vi "SGDA-Play Test.vi"(0 "StimChans":T1[](array[typedef]) {"Filter"."Stages"."IIR Filter"."Forward Coefficients" format="%.4f"; "Filter"."Stages"."IIR Filter"."Reverse Coefficients" format="%.4f"}, 1 "queue":refnum<queue>, 5 "Sampling rate (Hz)":dbl, 7 "Npts":i32, 11 "error in (no error)":errorcluster, 12 "Endpoint Config":T30[](array[typedef])) -> (15 "error out":errorcluster)   [LabVIEW 2020]
uses:
  Calibration VIs/Endpoint VIs/LV Source/Endpoint-Spec.ctl
  Calibration VIs/Endpoint VIs/LV Source/Endpoint-Modality.ctl
  Calibration VIs/Endpoint VIs/LV Source/Endpoint-Laterality.ctl
  Signal Synthesis VIs/3rd Generation/XControls/Stimulus Channel (G3)/Full Stimulus Channel Data.ctl
  Signal Synthesis VIs/3rd Generation/XControls/Waveform XControls/Waveform (G3)/Waveform Data.ctl
  Signal Synthesis VIs/3rd Generation/Waveform VIs/Waveform Enum (V3).ctl
  Signal Synthesis VIs/3rd Generation/XControls/Waveform XControls/Tone (G3)/Tone.Properties.ctl
  Signal Synthesis VIs/Waveform VIs/Pulse Train VIs/Pulse Train Params.ctl
  Signal Synthesis VIs/Waveform VIs/Pulse Train VIs/Pulse Polarity.ctl
  Signal Synthesis VIs/Waveform VIs/Pulse Train VIs/PT-Continuous State.ctl
  Signal Synthesis VIs/3rd Generation/Waveform VIs/Noise VIs/Noise (G3).ctl
  Signal Synthesis VIs/3rd Generation/Waveform VIs/Noise VIs/Noise (G3).Properties.ctl
  Signal Synthesis VIs/3rd Generation/Waveform VIs/Noise VIs/Noise (G3).Data.ctl
  Signal Synthesis VIs/Waveform VIs/File VIs/StimFile-Params.ctl
  Signal Synthesis VIs/Waveform VIs/FM Sweep VIs/FM Sweep Params.ctl
  Signal Synthesis VIs/Waveform VIs/Chirp Train VIs/Chirp Train.ctl
  Signal Synthesis VIs/Waveform VIs/Chirp Train VIs/Chirp Train Params.ctl
  Signal Synthesis VIs/Waveform VIs/Complex Tone VIs/CT-Params.ctl
  Signal Synthesis VIs/Waveform VIs/Complex Tone VIs/CT-Phase Enum.ctl
  Signal Synthesis VIs/Waveform VIs/Complex Tone VIs/CT-Runtime Data.ctl
  Signal Synthesis VIs/3rd Generation/XControls/Waveform XControls/FM Tone/Data.ctl
  Signal Synthesis VIs/3rd Generation/XControls/Waveform XControls/Vowel/Vowel.Properties.ctl
  Signal Synthesis VIs/3rd Generation/Waveform VIs/Ramp VIs/Ramp.Properties.ctl
  Signal Synthesis VIs/3rd Generation/XControls/Filter (G3)/Filter Data.ctl
  Signal Synthesis VIs/3rd Generation/XControls/Filter (G3)/Filter Type.ctl
  Signal Synthesis VIs/Filter VIs/Filter-Bandwidth Units.ctl
  Signal Synthesis VIs/Controls/Burst XCtl/Burst Data.ctl
  Signal Synthesis VIs/3rd Generation/XControls/Level (G3)/Level Data.ctl
  Signal Synthesis VIs/3rd Generation/XControls/Level (G3)/Level Units (G3).ctl
  Signal Synthesis VIs/3rd Generation/XControls/Advanced Options (G3)/Advanced Options (G3).ctl
  Signal Synthesis VIs/Modulation VIs/SAM VIs/SAM Params.ctl
  Signal Synthesis VIs/3rd Generation/Typedefs/Destination.ctl
  Type Defs/SGDA-Play Test Queue Data.ctl
  <vilib>/sound2/lvsound2.llb/Sound Data Format.ctl
  <vilib>/sound2/lvsound2.llb/Sampling Mode.ctl
  <vilib>/sound2/lvsound2.llb/Sound Output Write (DBL).vi
  Signal Synthesis VIs/3rd Generation/XControls/Filter (G3)/Filter (G3).xctl
  Signal Synthesis VIs/3rd Generation/XControls/Level (G3)/Level (G3).xctl
  Signal Synthesis VIs/Controls/Burst XCtl/Burst Control.xctl
  Signal Synthesis VIs/3rd Generation/XControls/Waveform XControls/Tone (G3)/Tone (G3).xctl
  Signal Synthesis VIs/3rd Generation/XControls/Waveform XControls/FM Tone/FM Tone.xctl
  Signal Synthesis VIs/3rd Generation/XControls/Waveform XControls/Waveform (G3)/Waveform (G3).xctl
  Signal Synthesis VIs/3rd Generation/XControls/Advanced Options (G3)/Advanced Options (G3).xctl
  Signal Synthesis VIs/3rd Generation/XControls/Stimulus Channel (G3)/Stimulus Channel (G3).xctl
  Signal Synthesis VIs/3rd Generation/XControls/Waveform XControls/Vowel/Vowel.xctl
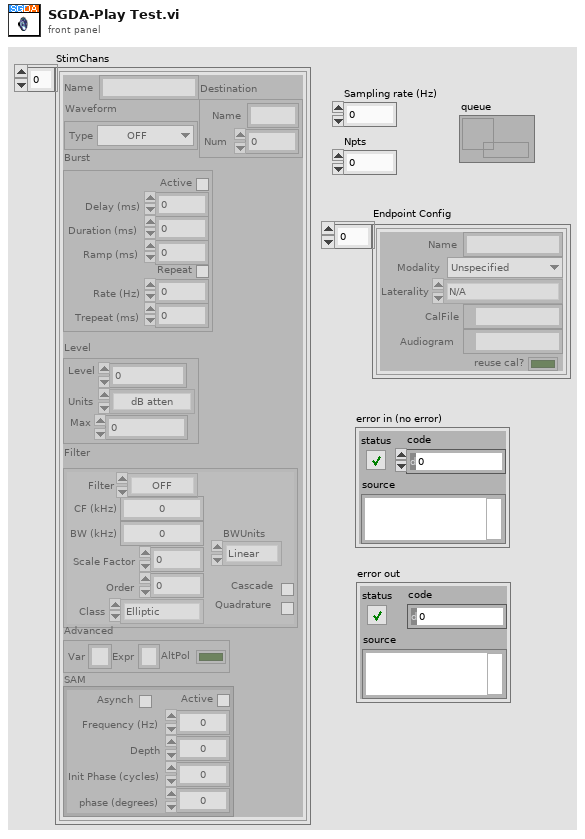
[diagram p1: front panel]
types:
  T1 = typedef "Stimulus Channel (G3).xctl/Full Stimulus Channel Data.ctl" = cluster{"Waveform":T2, "Filter":T21, "Burst":T24, "Level":T25, "Name":string, "Advanced":T27, "SAM":T28, "Destination":T29}
  T2 = typedef "Waveform (G3).xctl/Waveform Data.ctl" = cluster{"Type":T3, "Tone":T4, "Pulse Train":T5, "Noise":T8, "File":T11, "FMSweep":T12, "Chirp Train":T13, "Complex Tone":cluster{"Params":T15, "Data":T17}, "FM":T18, "Vowel":T19, "Ramp":T20}
  T3 = typedef "Waveform Enum (V3).ctl" = enum16{"OFF", "Tone", "Noise", "Pulse Train", "File", "FM Sweep", "Chirp Train", "Complex Tone", "FM Tone", "Vowel", "Ramp"}
  T4 = typedef "Tone (G3).xctl/Tone.Properties.ctl" = cluster{"Frequency (kHz)":dbl, "Phase (cycles)":dbl, "Random phase":bool}
  T5 = typedef "Pulse Train Params.ctl" = cluster{"Pulse width (us)":dbl, "Pulse rate (Hz)":dbl, "Gap (ms)":dbl, "Polarity":T6, "PT State":T7, "Asynch":bool}
  T6 = typedef "Pulse Polarity.ctl" = enum16{"POS", "NEG", "POS-NEG", "NEG-POS"}
  T7 = typedef "PT-Continuous State.ctl" = cluster{"Template":dbl[], "Nperiod":i32, "Index":i32, "Pulse Rate (Hz)":dbl, "Phase (cycles)":dbl, "Noff":i32}
  T8 = typedef "Noise (G3).ctl" = cluster{"Properties":T9, "Data":T10}
  T9 = typedef "Noise (G3).Properties.ctl" = cluster{"InvFilt":bool, "Aweight":bool, "Seed":i32, "Tokens":i32, "Brickwall":bool}
  T10 = typedef "Noise (G3).Data.ctl" = cluster{"TokenNum":i32}
  T11 = typedef "StimFile-Params.ctl" = cluster{"Filename":path, "Signal":dbl[], "Channel":i32, "stream":bool, "offset":i32, "nreps":i32, "loops":i32, "Randomize":bool, "order":i32[], "Seed":i32, "Tokens":i32}
  T12 = typedef "FM Sweep Params.ctl" = cluster{"Rate (oct/s)":dbl, "Fmin (Hz)":dbl, "Fmax (Hz)":dbl, "Ramp (ms)":dbl, "Linear":bool}
  T13 = typedef "Chirp Train.ctl" = cluster{"Params":T14, "Data":cluster{"WF":dbl[]}}
  T14 = typedef "Chirp Train Params.ctl" = cluster{"Fmin (kHz)":dbl, "Fmax (kHz)":dbl, "Compensate":bool, "Duration (ms)":dbl}
  T15 = typedef "CT-Params.ctl" = cluster{"F0 (Hz)":dbl, "Band":cluster{"Flow (Hz)":dbl, "Fhigh (Hz)":dbl}, "Phase":T16, "Min F0 (Hz)":dbl, "Max F0 (Hz)":dbl, "ContinRandPhase":bool, "Max peak factor":dbl, "Max mod depth":dbl, "MinHarmNum":i32, "MaxHarmNum":i32, "Level Mode":enum16{"per component", "overall rms"}, "% jitter":dbl}
  T16 = typedef "CT-Phase Enum.ctl" = enum16{"Cosine", "Random", "Alternating"}
  T17 = typedef "CT-Runtime Data.ctl" = cluster{"Ncomp":i32, "MinHarm":i32, "Phase":dbl[], "Amplitude":dbl[], "Npts/frame":i32, "Last F0":dbl, "Fmin":dbl, "Fmax":dbl, "Lslope":dbl, "randphase":bool, "overall rms":bool, "fmult":dbl[], "jittered":bool}
  T18 = typedef "FM Tone.xctl/Data.ctl" = cluster{"Carrier (kHz)":dbl, "ModRate (Hz)":dbl, "Depth (Hz)":dbl, "Phase (cycles)":dbl}
  T19 = typedef "Vowel.xctl/Vowel.Properties.ctl" = cluster{"Freqs":string, "Set level":enum16{"Total", "Per component"}, "Freq":dbl[], "weights":dbl[]}
  T20 = typedef "Ramp.Properties.ctl" = cluster{"Duration (ms)":dbl}
  T21 = typedef "Filter (G3).xctl/Filter Data.ctl" = cluster{"Type":T22, "CF (kHz)":dbl, "BW (kHz)":dbl, "Cascade":bool, "Quadrature":bool, "Scale Factor":dbl, "Stages":cluster{"IIR Filter":cluster{"filter structure":enum32{"IIR 2nd Order", "IIR 4th Order"}, "Reverse Coefficients":dbl[], "Forward Coefficients":dbl[]}, "State":dbl[]}[], "Class":enum16{"Elliptic", "Butterworth"}, "Order":i32, "BWUnits":T23}
  T22 = typedef "Filter (G3).xctl/Filter Type.ctl" = enum16{"OFF", "Lowpass", "Highpass", "Bandpass", "Bandstop"}
  T23 = typedef "Filter-Bandwidth Units.ctl" = enum16{"Linear", "Octaves", "Min-Max"}
  T24 = typedef "Burst Control.xctl/Burst Data.ctl" = cluster{"Active":bool, "Delay (ms)":dbl, "Duration (ms)":dbl, "Ramp (ms)":dbl, "Rate (Hz)":dbl, "Trepeat (ms)":dbl, "Repeat":bool}
  T25 = typedef "Level (G3).xctl/Level Data.ctl" = cluster{"Level":dbl, "Units":T26, "Max":dbl, "Data":cluster{"Multiplier":dbl, "Cal File":path, "Cal":cluster{"Freq (Hz)":dbl[], "Mag (dB SPL)":dbl[], "Phase (deg)":dbl[]}, "audiogram":path}}
  T26 = typedef "Level (G3).xctl/Level Units (G3).ctl" = enum16{"dB atten", "dB SPL", "dB re 1 Vrms", "dB V/Hz½", "mW", "dB HL", "Volts", "dB mW"}
  T27 = typedef "Advanced Options (G3).xctl/Advanced Options (G3).ctl" = cluster{"AltPol":bool, "Var":string, "Expr":string}
  T28 = typedef "SAM Params.ctl" = cluster{"Active":bool, "Frequency (Hz)":dbl, "Depth":dbl, "Init Phase (cycles)":dbl, "phase (degrees)":dbl, "Asynch":bool}
  T29 = typedef "Destination.ctl" = cluster{"Name":string, "Num":i32}
  T30 = typedef "Endpoint-Spec.ctl" = cluster{"Name":string, "Modality":T31, "Laterality":T32, "CalFile":path, "Audiogram":path, "reuse cal?":bool}
  T31 = typedef "Endpoint-Modality.ctl" = enum16{"Unspecified", "Acoustic", "Electric", "Optical"}
  T32 = typedef "Endpoint-Laterality.ctl" = enum16{"N/A", "Right", "Left"}
  T33 = typedef "Sound Data Format.ctl" = cluster{"sample rate (S/s)":dbl, "number of channels":i32, "bits per sample":i32}
  T34 = typedef "Sampling Mode.ctl" = i32
  T35 = typedef "Sound Output Task ID.ctl" = u32
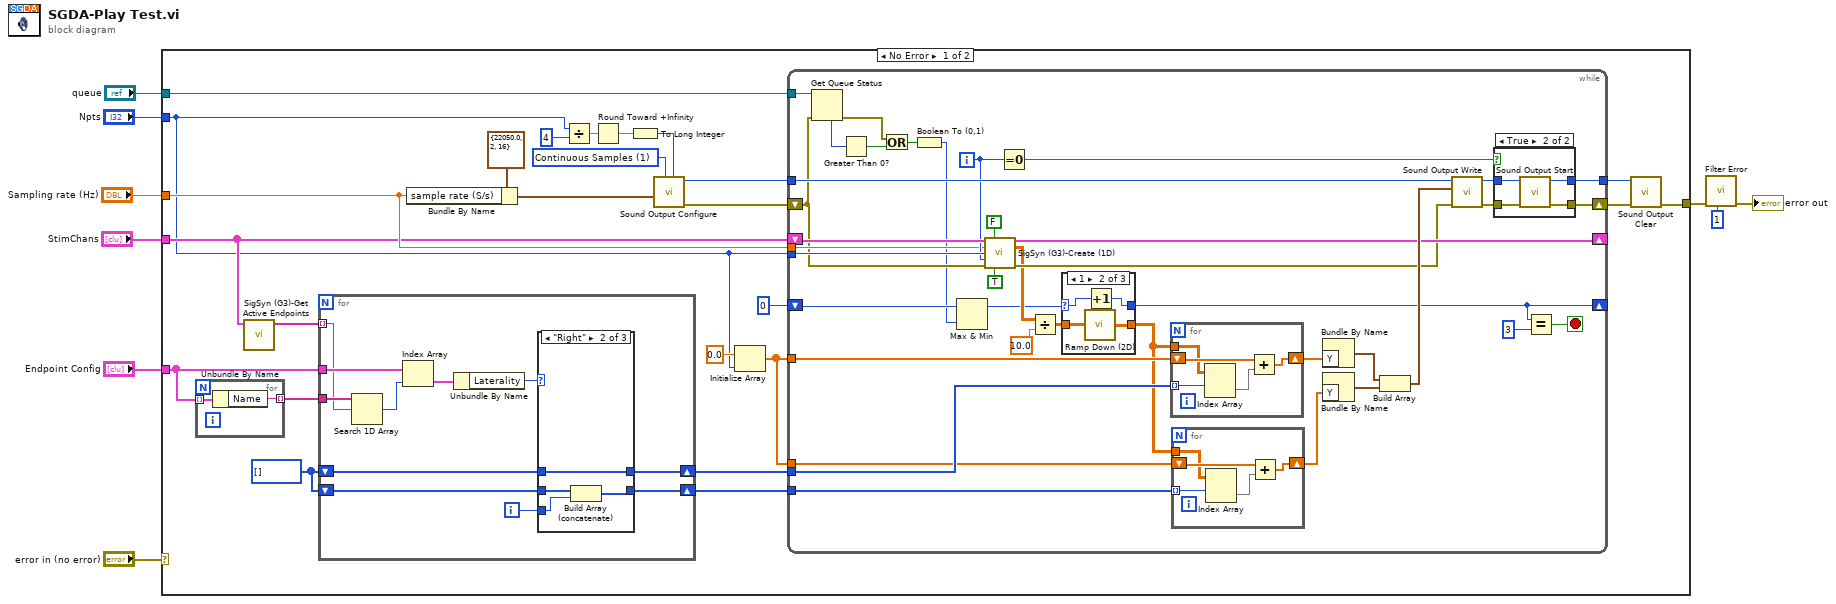
[diagram p0: block diagram]
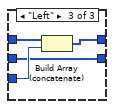
[diagram p3: hidden frame]
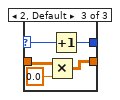
[diagram p5: hidden frame]
diagram:
  n1 = case shown="No Error" "error in (no error)" {
    selector: "error in (no error)" -> [_ w124]
    tunnel: [w19 w124] -> w8
    tunnel: "Sampling rate (Hz)" -> [w18 _]
    tunnel: "Endpoint Config" -> [w28 _]
    tunnel: "Npts" -> [w14 _]
    tunnel: "StimChans" -> [w17 _]
    tunnel: "queue" -> [w25 _]
    frame No Error {
      w26 = i32[] []
      w32 = T34 1 items=["Finite Samples", "Continuous Samples"] ("sample mode")
      n2 = for {
        tunnel: w28 -> [w36] mode=indexing
        tunnel: [w35] -> w29 mode=indexing
        n3 = Unbundle By Name(w36) -> ("Name"=w35:string)
      }
      n4 = call "SigSyn (G3)-Get Active Endpoints.vi"("StimChans In"=w17) -> ("Active Endpoints"=w16:string[])  [unwired: 9 in, 1 out]
      n5 = for {
        tunnel: w29 -> [w47]
        tunnel: w28 -> [w46]
        tunnel: w16 -> [w43] mode=indexing
        shift-right: [w37] -> w23
        shift-left: w26 -> [w41]
        shift-right: [w38] -> w22
        shift-left: w26 -> [w40]
        i -> [w39]
        n6 = Search 1D Array(1D array=w47, element=w43) -> (index of element=w45:i32)  [unwired: 1 in]
        n7 = Index Array(array=w46, index=w45) -> (element=w44:T30)
        n8 = Unbundle By Name(w44) -> ("Laterality"=w42:T32)
        n9 = case shown="\"Right\"" w42 {
          tunnel: w41 -> [w49 w50 w56]
          tunnel: w40 -> [w48 w53 w54]
          tunnel: w39 -> [_ w52 w57]
          tunnel: [w48 w51 w54] -> w38
          tunnel: [w49 w50 w55] -> w37
          frame "N/A", Default {
          }
          frame "Right" {
            n10 = Build Array (concatenate)(w53, w52) -> (w51:i32[])
          }
          frame "Left" {
            n11 = Build Array (concatenate)(w56, w57) -> (w55:i32[])
          }
        }
      }
      n12 = Bundle By Name(cluster=T33 {"sample rate (S/s)"=22050.0, "number of channels"=2, "bits per sample"=16} ("sound format"), "sample rate (S/s)"=w18) -> (w33:T33)
      n13 = Divide(x=w14, y=4) -> (x/y=w12:dbl)
      n14 = Round Toward +Infinity(x=w12) -> (ceil(x): smallest int >= x=w11:dbl)
      n15 = To Long Integer(number=w11) -> (32bit integer=w10:i32)
      n16 = call <vilib>:"Sound Output Configure.vi"("number of samples/ch"=w10, "sample mode"=w32, "sound format"=w33) -> ("error out"=w31:errorcluster, "task ID"=w30:T35)  [unwired: 7 in]
      n17 = Initialize Array(0.0, w14) -> (w24:dbl[])
      n18 = while {
        tunnel: w30 -> [w96]
        tunnel: w25 -> [w76]
        shift-right: [w86] -> _
        shift-left: w17 -> [w87]
        tunnel: w24 -> [w84]
        tunnel: w24 -> [w79]
        tunnel: w23 -> [w83]
        tunnel: w22 -> [w80]
        tunnel: [w77] -> w21
        tunnel: w14 -> [w72]
        tunnel: w18 -> [w70]
        shift-right: [w60] -> _
        shift-left: 0 -> [w63]
        shift-right: [w65] -> w20
        shift-left: w31 -> [w64]
        i -> [w71]
        stop <- w58 stop-if-true
        n19 = Get Queue Status(queue=w76, error in (no error)=w64) -> (error out=w74:errorcluster, # elements in queue=w75:i32)  [unwired: 1 in, 6 out]
        n20 = Greater Than 0?(x=w75) -> (x > 0?=w69:bool)
        n21 = Or(x=w74, y=w69) -> (x .or. y?=w66:bool)
        n22 = Boolean To (0,1)(Boolean=w66) -> (0, 1=w62:i16)
        n23 = Max & Min(x=w63, y=w62) -> (max(x,y)=w61:i32)  [unwired: 1 out]
        n24 = call "SigSyn (G3)-Create (1D).vi"("StimChans In"=w87, "Apply multipliers? (F)"=FALSE, "Sampling Rate (Hz)"=w70, "Npts"=w72, "Rep Num"=w71, "error in (no error)"=w64, "Zero unused (F)"=TRUE) -> ("StimChans Out"=w86:T1[], "Waveform"=w81:dbl[][], "error out"=w85:errorcluster)  [unwired: 5 in, 1 out]
        n25 = Equal To 0?(x=w71) -> (x = 0?=w90:bool)
        n26 = Divide(x=w81, y=10.0) -> (x/y=w68:dbl[][])
        n27 = case shown="1" w61 {
          selector: w61 -> [w97 w100 w104]
          tunnel: w68 -> [w98 w102 w107]
          tunnel: [w98 w101 w106] -> w67
          tunnel: [w97 w99 w103] -> w60
          frame 0 {
          }
          frame 1 {
            n28 = call "Ramp Down (2D).vi"("Array"=w102) -> ("Ramped array"=w101:dbl[][])  [unwired: 4 in]
            n29 = Increment(x=w100) -> (x+1=w99:i32)
          }
          frame 2, Default {
            n30 = Multiply(x=w107, y=0.0) -> (x*y=w106:dbl[][])
            n31 = Increment(x=w104) -> (x+1=w103:i32)
          }
        }
        n32 = for {
          tunnel: w67 -> [w115]
          tunnel: w83 -> [w116] mode=indexing
          shift-right: [w113] -> w82
          shift-left: w84 -> [w117]
          n33 = Index Array(array=w115, index (row)=w116) -> (element=w114:dbl[])  [unwired: 1 in]
          n34 = Add(x=w117, y=w114) -> (x+y=w113:dbl[])
        }
        n35 = for {
          tunnel: w67 -> [w110]
          tunnel: w80 -> [w111] mode=indexing
          shift-right: [w108] -> w78
          shift-left: w79 -> [w112]
          n36 = Index Array(array=w110, index (row)=w111) -> (element=w109:dbl[])  [unwired: 1 in]
          n37 = Add(x=w112, y=w109) -> (x+y=w108:dbl[])
        }
        n38 = Bundle By Name("Y"=w82) -> (w93:waveform(dbl))  [unwired: 1 in]
        n39 = Bundle By Name("Y"=w78) -> (w92:waveform(dbl))  [unwired: 1 in]
        n40 = Build Array(w93, w92) -> (w91:waveform(dbl)[])
        n41 = call-poly <vilib>:"Sound Output Write.vi"("error in (no error)"=w85, "data"=w91, "task ID"=w96) -> ("error out"=w94:errorcluster, "task ID out"=w95:T35)  [unwired: 7 in]
        n42 = case shown="True" w90 {
          tunnel: w95 -> [w118 w123]
          tunnel: w94 -> [w119 w122]
          tunnel: [w119 w121] -> w65
          tunnel: [w118 w120] -> w77
          frame False {
          }
          frame True {
            n43 = call <vilib>:"Sound Output Start.vi"("error in (no error)"=w122, "task ID"=w123) -> ("error out"=w121:errorcluster, "task ID out"=w120:T35)  [unwired: 8 in]
          }
        }
        n44 = Equal?(x=w60, y=3) -> (x = y?=w58:bool)
      }
      n45 = call <vilib>:"Sound Output Clear.vi"("error in (no error)"=w20, "task ID"=w21) -> ("error out"=w19:errorcluster)  [unwired: 9 in]
    }
    frame Error {
    }
  }
  n46 = call "Filter Error.vi"("error in (no error)"=w8, "code to ignore"=1) -> ("error out"=→"error out":errorcluster)  [unwired: 9 in]
